vi "EnumDevices.vi"(5 "nLayerType":u32=1, 11 "error in (no error)":errorcluster caption="错误输入（无错误）") -> (4 "function return":i32, 6 "nDeviceNumReturn":u32, 8 "GigEDeviceArray":T2(array[cluster]), 10 "U3VDeviceArray":T1(array[cluster]), 15 "error out":errorcluster caption="错误输出")   [LabVIEW 2011, in "MvCameraControl.lvlib"]
uses:
  MvCameraControl.lvlib
  x86/MvCameraPatch.dll
panel:
  in  "U3VDevice":T3
  in  "GigEDevice":T4
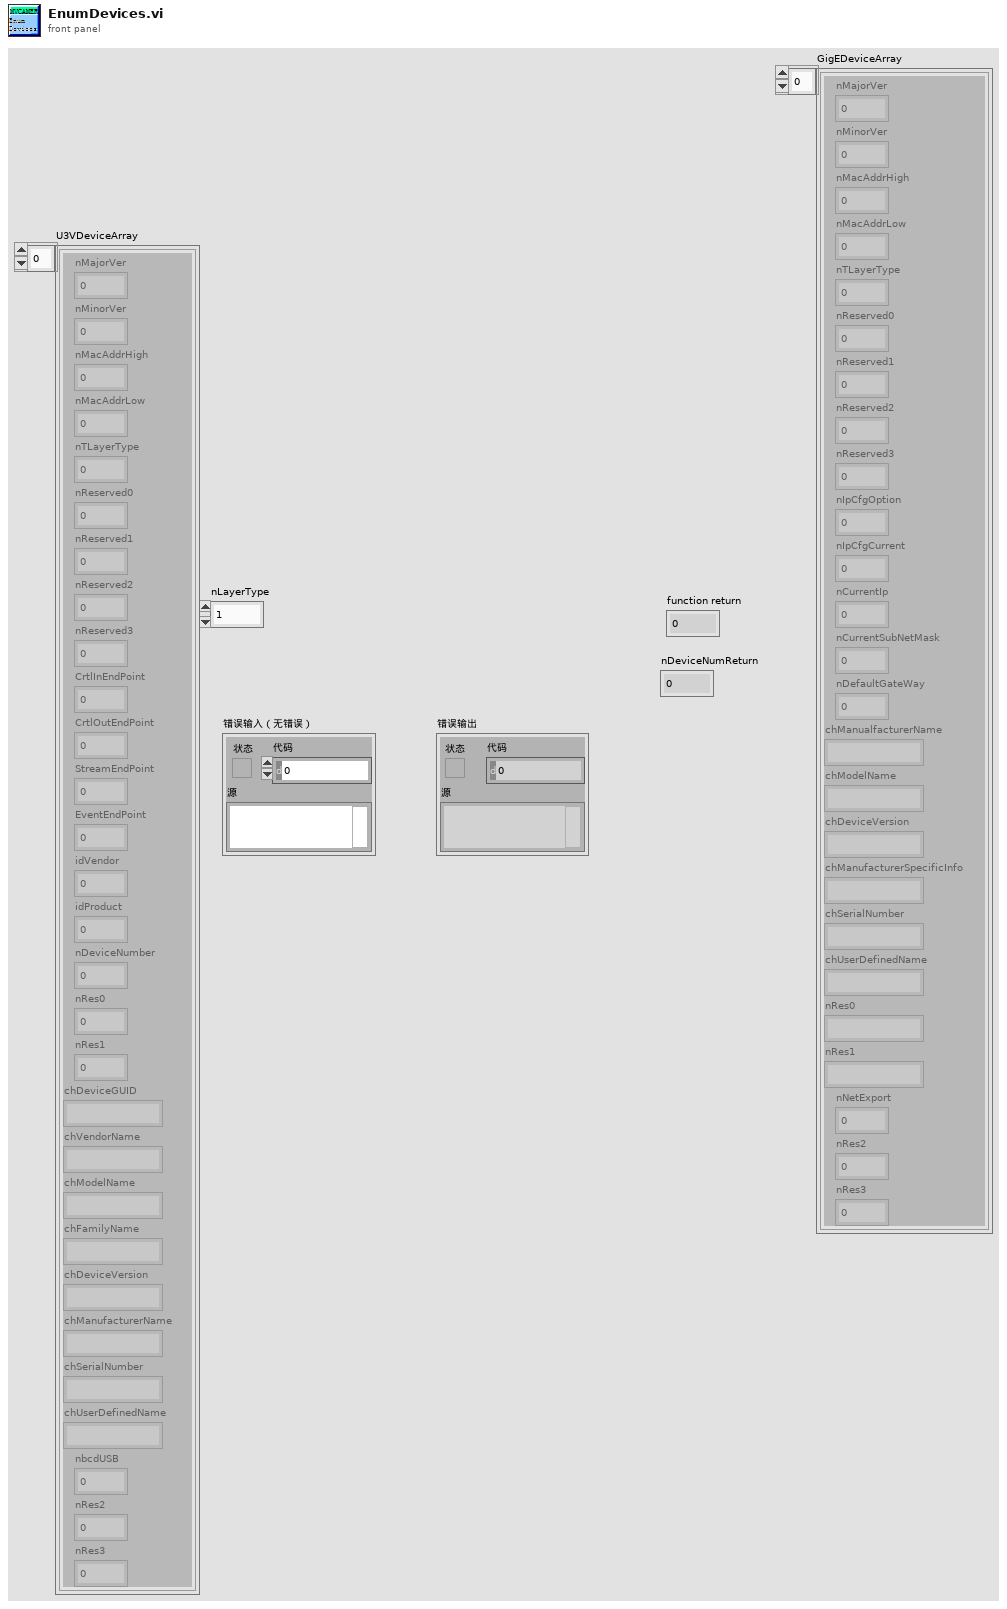
[diagram p1: front panel]
types:
  T1 = cluster{"nMajorVer":u16, "nMinorVer":u16, "nMacAddrHigh":u32, "nMacAddrLow":u32, "nTLayerType":u32, "nReserved0":u32, "nReserved1":u32, "nReserved2":u32, "nReserved3":u32, "CrtlInEndPoint":u8, "CrtlOutEndPoint":u8, "StreamEndPoint":u8, "EventEndPoint":u8, "idVendor":u16, "idProduct":u16, "nDeviceNumber":u32, "nRes0":u32, "nRes1":u32, "chDeviceGUID":string, "chVendorName":string, "chModelName":string, "chFamilyName":string, "chDeviceVersion":string, "chManufacturerName":string, "chSerialNumber":string, "chUserDefinedName":string, "nbcdUSB":u32, "nRes2":u32, "nRes3":u32}[]
  T2 = cluster{"nMajorVer":u16, "nMinorVer":u16, "nMacAddrHigh":u32, "nMacAddrLow":u32, "nTLayerType":u32, "nReserved0":u32, "nReserved1":u32, "nReserved2":u32, "nReserved3":u32, "nIpCfgOption":u32, "nIpCfgCurrent":u32, "nCurrentIp":u32, "nCurrentSubNetMask":u32, "nDefaultGateWay":u32, "chManualfacturerName":string, "chModelName":string, "chDeviceVersion":string, "chManufacturerSpecificInfo":string, "chSerialNumber":string, "chUserDefinedName":string, "nRes0":string, "nRes1":string, "nNetExport":u32, "nRes2":u32, "nRes3":u32}[]
  T3 = cluster{"nMajorVer":u16, "nMinorVer":u16, "nMacAddrHigh":u32, "nMacAddrLow":u32, "nTLayerType":u32, "nReserved0":u32, "nReserved1":u32, "nReserved2":u32, "nReserved3":u32, "CrtlInEndPoint":u8, "CrtlOutEndPoint":u8, "StreamEndPoint":u8, "EventEndPoint":u8, "idVendor":u16, "idProduct":u16, "nDeviceNumber":u32, "nRes0":u32, "nRes1":u32, "chDeviceGUID":string, "chVendorName":string, "chModelName":string, "chFamilyName":string, "chDeviceVersion":string, "chManufacturerName":string, "chSerialNumber":string, "chUserDefinedName":string, "nbcdUSB":u32, "nRes2":u32, "nRes3":u32}
  T4 = cluster{"nMajorVer":u16, "nMinorVer":u16, "nMacAddrHigh":u32, "nMacAddrLow":u32, "nTLayerType":u32, "nReserved0":u32, "nReserved1":u32, "nReserved2":u32, "nReserved3":u32, "nIpCfgOption":u32, "nIpCfgCurrent":u32, "nCurrentIp":u32, "nCurrentSubNetMask":u32, "nDefaultGateWay":u32, "chManualfacturerName":string, "chModelName":string, "chDeviceVersion":string, "chManufacturerSpecificInfo":string, "chSerialNumber":string, "chUserDefinedName":string, "nRes0":string, "nRes1":string, "nNetExport":u32, "nRes2":u32, "nRes3":u32}
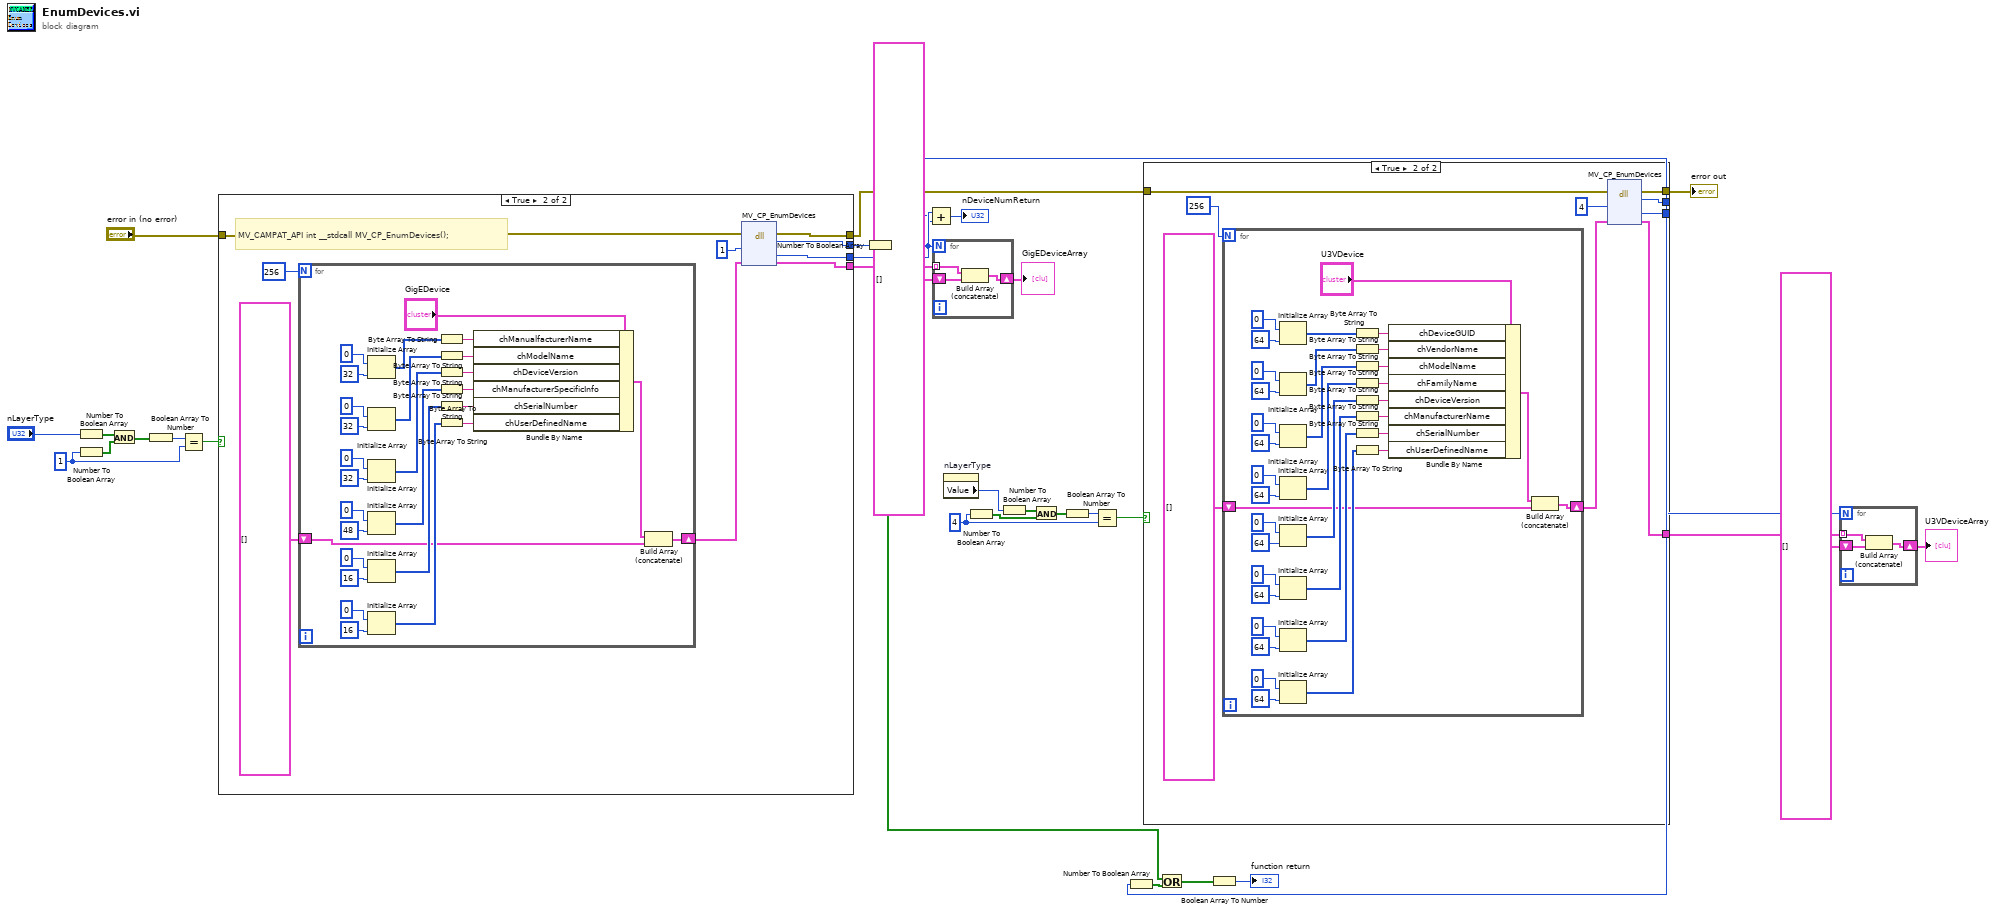
[diagram p0: block diagram]
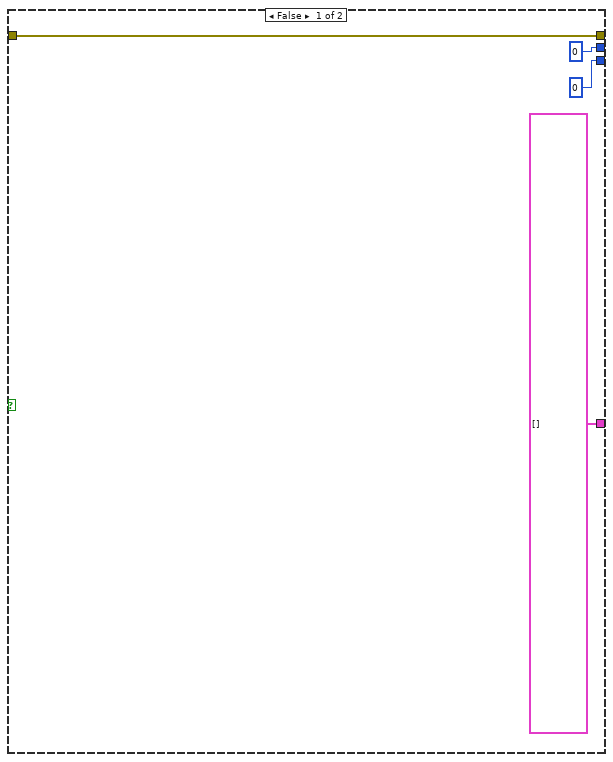
[diagram p2: hidden frame]
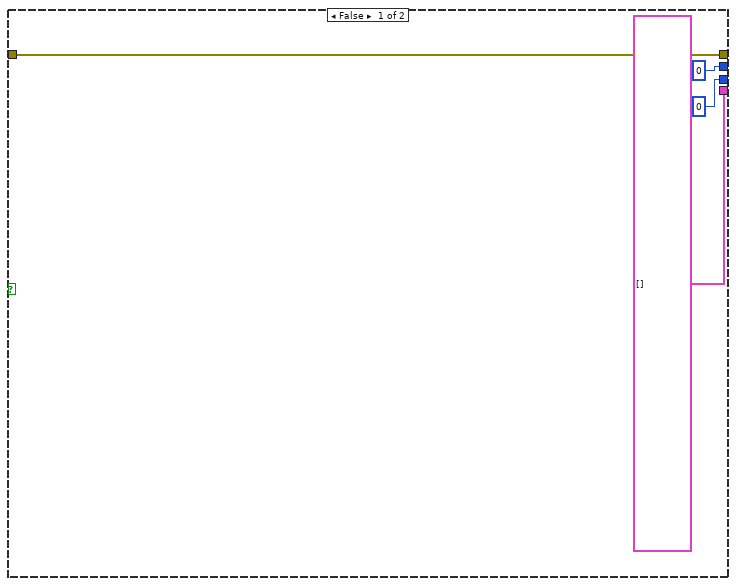
[diagram p3: hidden frame]
diagram:
  w20 = u32 4 ("数字")
  w28 = u32 1 ("数字")
  n1 = Number To Boolean Array(number="nLayerType") -> (Boolean array=w32:bool[])
  n2 = Number To Boolean Array(number=w28) -> (Boolean array=w31:bool[])
  n3 = And(x=w32, y=w31) -> (x .and. y?=w30:bool[])
  n4 = Boolean Array To Number(Boolean array=w30) -> (number=w29:u32)
  n5 = Equal?(x=w29, y=w28) -> (x = y?=w27:bool)
  n6 = case shown="True" w27 {
    tunnel: [0 ("返回类型") w42] -> w16
    tunnel: [u32 0 ("nDeviceNumReturn") w41] -> w9
    tunnel: "error in (no error)" -> [w34 w40]
    tunnel: [w34 w39] -> w11
    tunnel: [T2 [] ("DeviceInfoArray") w37] -> w6
    frame False {
    }
    frame True {
      # "MV_CAMPAT_API int __stdcall MV_CP_EnumDevices();"
      n7 = for {
        N: 256 -> [_]
        shift-right: [w48] -> w45
        shift-left: T2 [] -> [w46]
        n8 = Initialize Array(u8 0 ("元素"), 32 ("维数大小")) -> (w57:u8[])
        n9 = Initialize Array(u8 0 ("元素"), 32 ("维数大小")) -> (w60:u8[])
        n10 = Initialize Array(u8 0 ("元素"), 32 ("维数大小")) -> (w49:u8[])
        n11 = Initialize Array(u8 0 ("元素"), 48 ("维数大小")) -> (w54:u8[])
        n12 = Initialize Array(u8 0 ("元素"), 16 ("维数大小")) -> (w68:u8[])
        n13 = Initialize Array(u8 0 ("元素"), 16 ("维数大小")) -> (w65:u8[])
        n14 = Byte Array To String(unsigned byte array=w57) -> (string=w69:string)
        n15 = Byte Array To String(unsigned byte array=w60) -> (string=w70:string)
        n16 = Byte Array To String(unsigned byte array=w49) -> (string=w50:string)
        n17 = Byte Array To String(unsigned byte array=w54) -> (string=w71:string)
        n18 = Byte Array To String(unsigned byte array=w68) -> (string=w72:string)
        n19 = Byte Array To String(unsigned byte array=w65) -> (string=w73:string)
        n20 = Bundle By Name(cluster="GigEDevice", "chManualfacturerName"=w69, "chModelName"=w70, "chDeviceVersion"=w50, "chManufacturerSpecificInfo"=w71, "chSerialNumber"=w72, "chUserDefinedName"=w73) -> (w47:T4)
        n21 = Build Array (concatenate)(w47, w46) -> (w48:T2)
      }
      n22 = dll-call lib="MvCameraPatch.dll" fn="MV_CP_EnumDevices"(error in=w40, "nLayerType"=u32 1, "DeviceInfoArray"=w45) -> (error out=w39:errorcluster, "返回类型"=w42:i32, "nDeviceNumReturn"=w41:u32, "DeviceInfoArray"=w37:T2)  [unwired: 4 in, 1 out]
    }
  }
  n23 = Number To Boolean Array(number=w16) -> (Boolean array=w15:bool[])
  n24 = for {
    N: w9 -> [_]
    tunnel: w6 -> [w76] mode=indexing
    shift-right: [w74] -> w4
    shift-left: T2 [] -> [w75]
    n25 = Build Array (concatenate)(w76, w75) -> (w74:T2)
  }
  "GigEDeviceArray" <- w4
  n26 = property on="nLayerType" class="DigNum (strict)"() -> ("Value"=w7:u32)  [unwired: 2 in, 2 out]
  n27 = Number To Boolean Array(number=w20) -> (Boolean array=w23:bool[])
  n28 = Number To Boolean Array(number=w7) -> (Boolean array=w24:bool[])
  n29 = And(x=w24, y=w23) -> (x .and. y?=w22:bool[])
  n30 = Boolean Array To Number(Boolean array=w22) -> (number=w21:u32)
  n31 = Equal?(x=w21, y=w20) -> (x = y?=w19:bool)
  n32 = case shown="True" w19 {
    tunnel: [u32 0 ("nDeviceNumReturn") w88] -> w8
    tunnel: [0 ("返回类型") w87] -> w17
    tunnel: w11 -> [w78 w86]
    tunnel: [w78 w85] -> w10
    tunnel: [T1 [] w81] -> w3
    frame False {
    }
    frame True {
      n33 = for {
        N: 256 -> [_]
        shift-right: [w90] -> w83
        shift-left: T1 [] -> [w92]
        n34 = Initialize Array(u8 0 ("元素"), 64 ("维数大小")) -> (w96:u8[])
        n35 = Initialize Array(u8 0 ("元素"), 64 ("维数大小")) -> (w100:u8[])
        n36 = Initialize Array(u8 0 ("元素"), 64 ("维数大小")) -> (w103:u8[])
        n37 = Initialize Array(u8 0 ("元素"), 64 ("维数大小")) -> (w106:u8[])
        n38 = Initialize Array(u8 0 ("元素"), 64 ("维数大小")) -> (w109:u8[])
        n39 = Initialize Array(u8 0 ("元素"), 64 ("维数大小")) -> (w112:u8[])
        n40 = Initialize Array(u8 0 ("元素"), 64 ("维数大小")) -> (w119:u8[])
        n41 = Initialize Array(u8 0 ("元素"), 64 ("维数大小")) -> (w124:u8[])
        n42 = Byte Array To String(unsigned byte array=w96) -> (string=w97:string)
        n43 = Byte Array To String(unsigned byte array=w100) -> (string=w113:string)
        n44 = Byte Array To String(unsigned byte array=w103) -> (string=w114:string)
        n45 = Byte Array To String(unsigned byte array=w106) -> (string=w115:string)
        n46 = Byte Array To String(unsigned byte array=w109) -> (string=w116:string)
        n47 = Byte Array To String(unsigned byte array=w112) -> (string=w120:string)
        n48 = Byte Array To String(unsigned byte array=w119) -> (string=w121:string)
        n49 = Byte Array To String(unsigned byte array=w124) -> (string=w125:string)
        n50 = Bundle By Name(cluster="U3VDevice", "chDeviceGUID"=w97, "chVendorName"=w113, "chModelName"=w114, "chFamilyName"=w115, "chDeviceVersion"=w116, "chManufacturerName"=w120, "chSerialNumber"=w121, "chUserDefinedName"=w125) -> (w91:T3)
        n51 = Build Array (concatenate)(w91, w92) -> (w90:T1)
      }
      n52 = dll-call lib="MvCameraPatch.dll" fn="MV_CP_EnumDevices"(error in=w86, "nLayerType"=u32 4, "DeviceInfoArray"=w83) -> (error out=w85:errorcluster, "返回类型"=w87:i32, "nDeviceNumReturn"=w88:u32, "DeviceInfoArray"=w81:T1)  [unwired: 4 in, 1 out]
    }
  }
  "error out" <- w10
  n53 = Add(x=w9, y=w8) -> (x+y=→"nDeviceNumReturn":u32)
  n54 = Number To Boolean Array(number=w17) -> (Boolean array=w14:bool[])
  n55 = Or(x=w15, y=w14) -> (x .or. y?=w13:bool[])
  n56 = Boolean Array To Number(Boolean array=w13) -> (number=→"function return":u32)
  n57 = for {
    N: w8 -> [_]
    tunnel: w3 -> [w128] mode=indexing
    shift-right: [w126] -> w1
    shift-left: T1 [] -> [w127]
    n58 = Build Array (concatenate)(w128, w127) -> (w126:T1)
  }
  "U3VDeviceArray" <- w1
